vi "Clusters.vi"() -> ()   [LabVIEW 2022 SP3]
panel:
  out "First Name":string
  in  "Cluster":T1
  out "Female":bool
  out "Age 2":dbl
  out "Last Name 2":string
  out "First Name 2":string
  # "Male"
  # "Male"
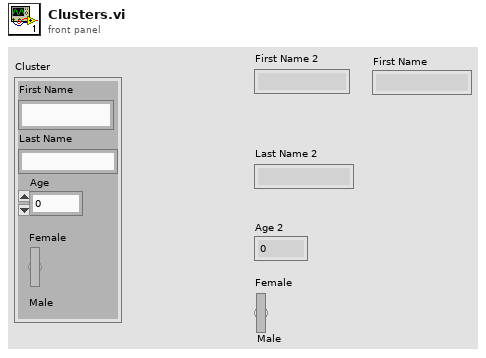
[diagram p1: front panel]
types:
  T1 = cluster{"First Name":string, "Last Name":string, "Age":dbl, "Female":bool}
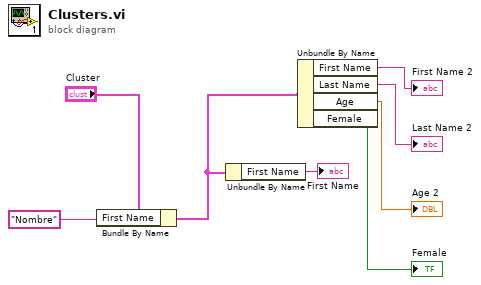
[diagram p0: block diagram]
diagram:
  n1 = Bundle By Name(cluster="Cluster", "First Name"="Nombre") -> (w2:T1)
  n2 = Unbundle By Name(w2) -> ("First Name"=→"First Name":string)
  n3 = Unbundle By Name "Unbundle By Name"(w2) -> ("First Name"=→"First Name 2":string, "Last Name"=→"Last Name 2":string, "Age"=→"Age 2":dbl, "Female"=→"Female":bool)
